vi "Refname to String (Drive).vi"(1 "Enum":T1) -> (0 "resulting string":string)   [LabVIEW 2016, in "Huskie Swerve.lvlib"]
uses:
  Huskie Swerve.lvlib
  Drive Motors.ctl
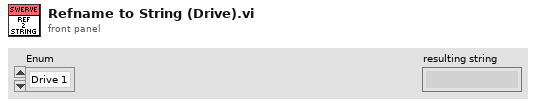
[diagram p1: front panel]
types:
  T1 = typedef "Huskie Swerve.lvlib/Drive Motors.ctl" = enum16{"Drive 1", "Drive 2", "Drive 3", "Drive 4"}
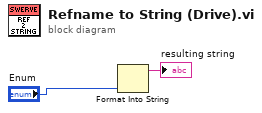
[diagram p0: block diagram]
diagram:
  n1 = Format Into String("Enum") -> (resulting string=→"resulting string":string)  [unwired: 3 in, 1 out]
